vi "Configure Measurements Function.vi"(7 "Operation (0: Meas Histogram Function)":i32(ring) items=["Meas Histogram Function", "Meas Trend Function"], 8 "error in (no error)":errorcluster, 9 "Meas Function (0: Measurement 1)":i32(ring) items=["Measurement 1", "Measurement 2", "Measurement 3", "Measurement 4", "Measurement 5"], 10 "Channel (1: Function 1)":i32(ring)=1 items=["Function 1"=1, "Function 2"=2, "Function 3"=3, "Function 4"=4, "Function 5"=5, "Function 6"=6, "Function 7"=7, "Function 8"=8, "Function 9"=9, "Function 10"=10, "Function 11"=11, "Function 12"=12, "Function 13"=13, "Function 14"=14, "Function 15"=15, "Function 16"=16], 11 "VISA resource name":refnum<visa-resource-name>) -> (0 "error out":errorcluster, 3 "VISA resource name out":refnum<visa-resource-name>)   [LabVIEW 2013, in "Agilent 90000 Series.lvlib"]
doc: "Sets up a measurement function to a measurement."
uses:
  Agilent 90000 Series.lvlib
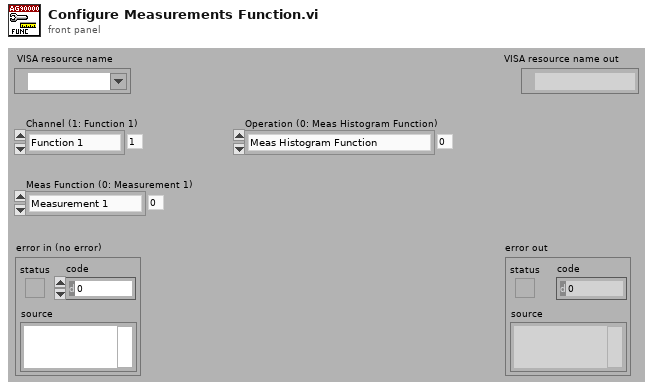
[diagram p1: front panel]
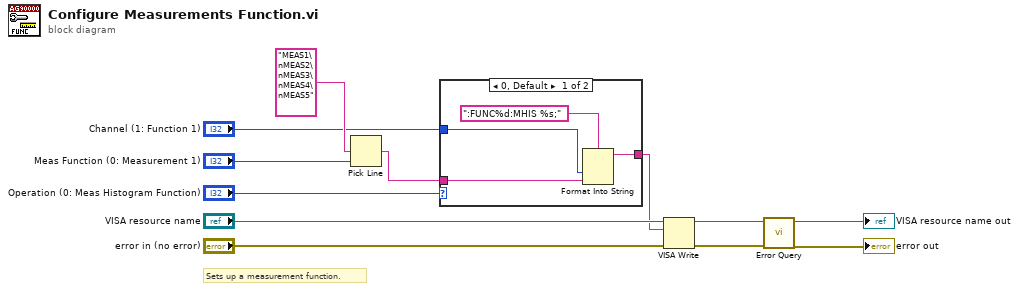
[diagram p0: block diagram]
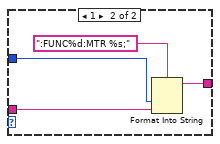
[diagram p2: hidden frame]
diagram:
  # "Sets up a measurement function."
  n1 = Pick Line(multi-line string="MEAS1\nMEAS2\nMEAS3\nMEAS4\nMEAS5", line index="Meas Function (0: Measurement 1)") -> (output string=w3:string)  [unwired: 1 out]
  n2 = case shown="0, Default" "Operation (0: Meas Histogram Function)" {
    tunnel: w3 -> [w16 w18]
    tunnel: "Channel (1: Function 1)" -> [w15 w19]
    tunnel: [w13 w17] -> w1
    frame 0, Default {
      n3 = Format Into String(format string=":FUNC%d:MHIS %s;", w15, w16) -> (resulting string=w13:string)  [unwired: 2 in, 1 out]
    }
    frame 1 {
      n4 = Format Into String(format string=":FUNC%d:MTR %s;", w19, w18) -> (resulting string=w17:string)  [unwired: 2 in, 1 out]
    }
  }
  n5 = VISA Write(VISA resource name="VISA resource name", write buffer=w1, error in (no error)="error in (no error)") -> (VISA resource name out=w8:refnum<visa-resource-name>, error out=w7:errorcluster)  [unwired: 1 out]
  n6 = call "Error Query.vi"("error in (no error)"=w7, "VISA resource name"=w8) -> ("error out"=→"error out":errorcluster, "VISA resource name out"=→"VISA resource name out":refnum<visa-resource-name>)  [unwired: 8 out]
